vi "fromFiles.vi"(0 "MagAnalysis_Online in":refnum<class "MagAnalysis_Online.lvclass">, 1 "SubscriberCluster":T1, 2 "Clibration":T7, 5 "Images":T6, 7 "BGImages":T3, 9 "data":T5, 11 "error in (no error)":errorcluster, 12 "Numeric 3":i32) -> (3 "OK":bool[](array[boolean]), 4 "MagAnalysis_Online out":refnum<class "MagAnalysis_Online.lvclass">, 6 "ROI":T11, 8 "new ROI":bool, 10 "spec cluster":cluster{dbl[], dbl[]}, 13 "Numeric 2":u32, 14 "change from file":dbl, 15 "Numeric":dbl)   [LabVIEW 2011, in "MagAnalysis_Online.lvclass"]
uses:
  MagAnalysis_Online.lvclass
  SubVis/ROIStartfromCam_typdef.ctl
  SubVis/ScreenCam_TypDEf.ctl
  SubVis/ROIInfo_TypDef.ctl
  calib_Sub_Typdef.ctl
  Calib_Typdef.ctl
  <vilib>/vision/Image Controls.llb/IMAQ Image.ctl
  analysis_data_typdef.ctl
  SubVis/dataTypdef.ctl
  bgImages_tyudef.ctl
  Interface/GUI_Template/GUI_master/tcp new data cluster.ctl
  Interface/GUI_Template/GUI_master/tcp_new_data_event.ctl
  shared/SubscriberCluster_TypDEf.ctl
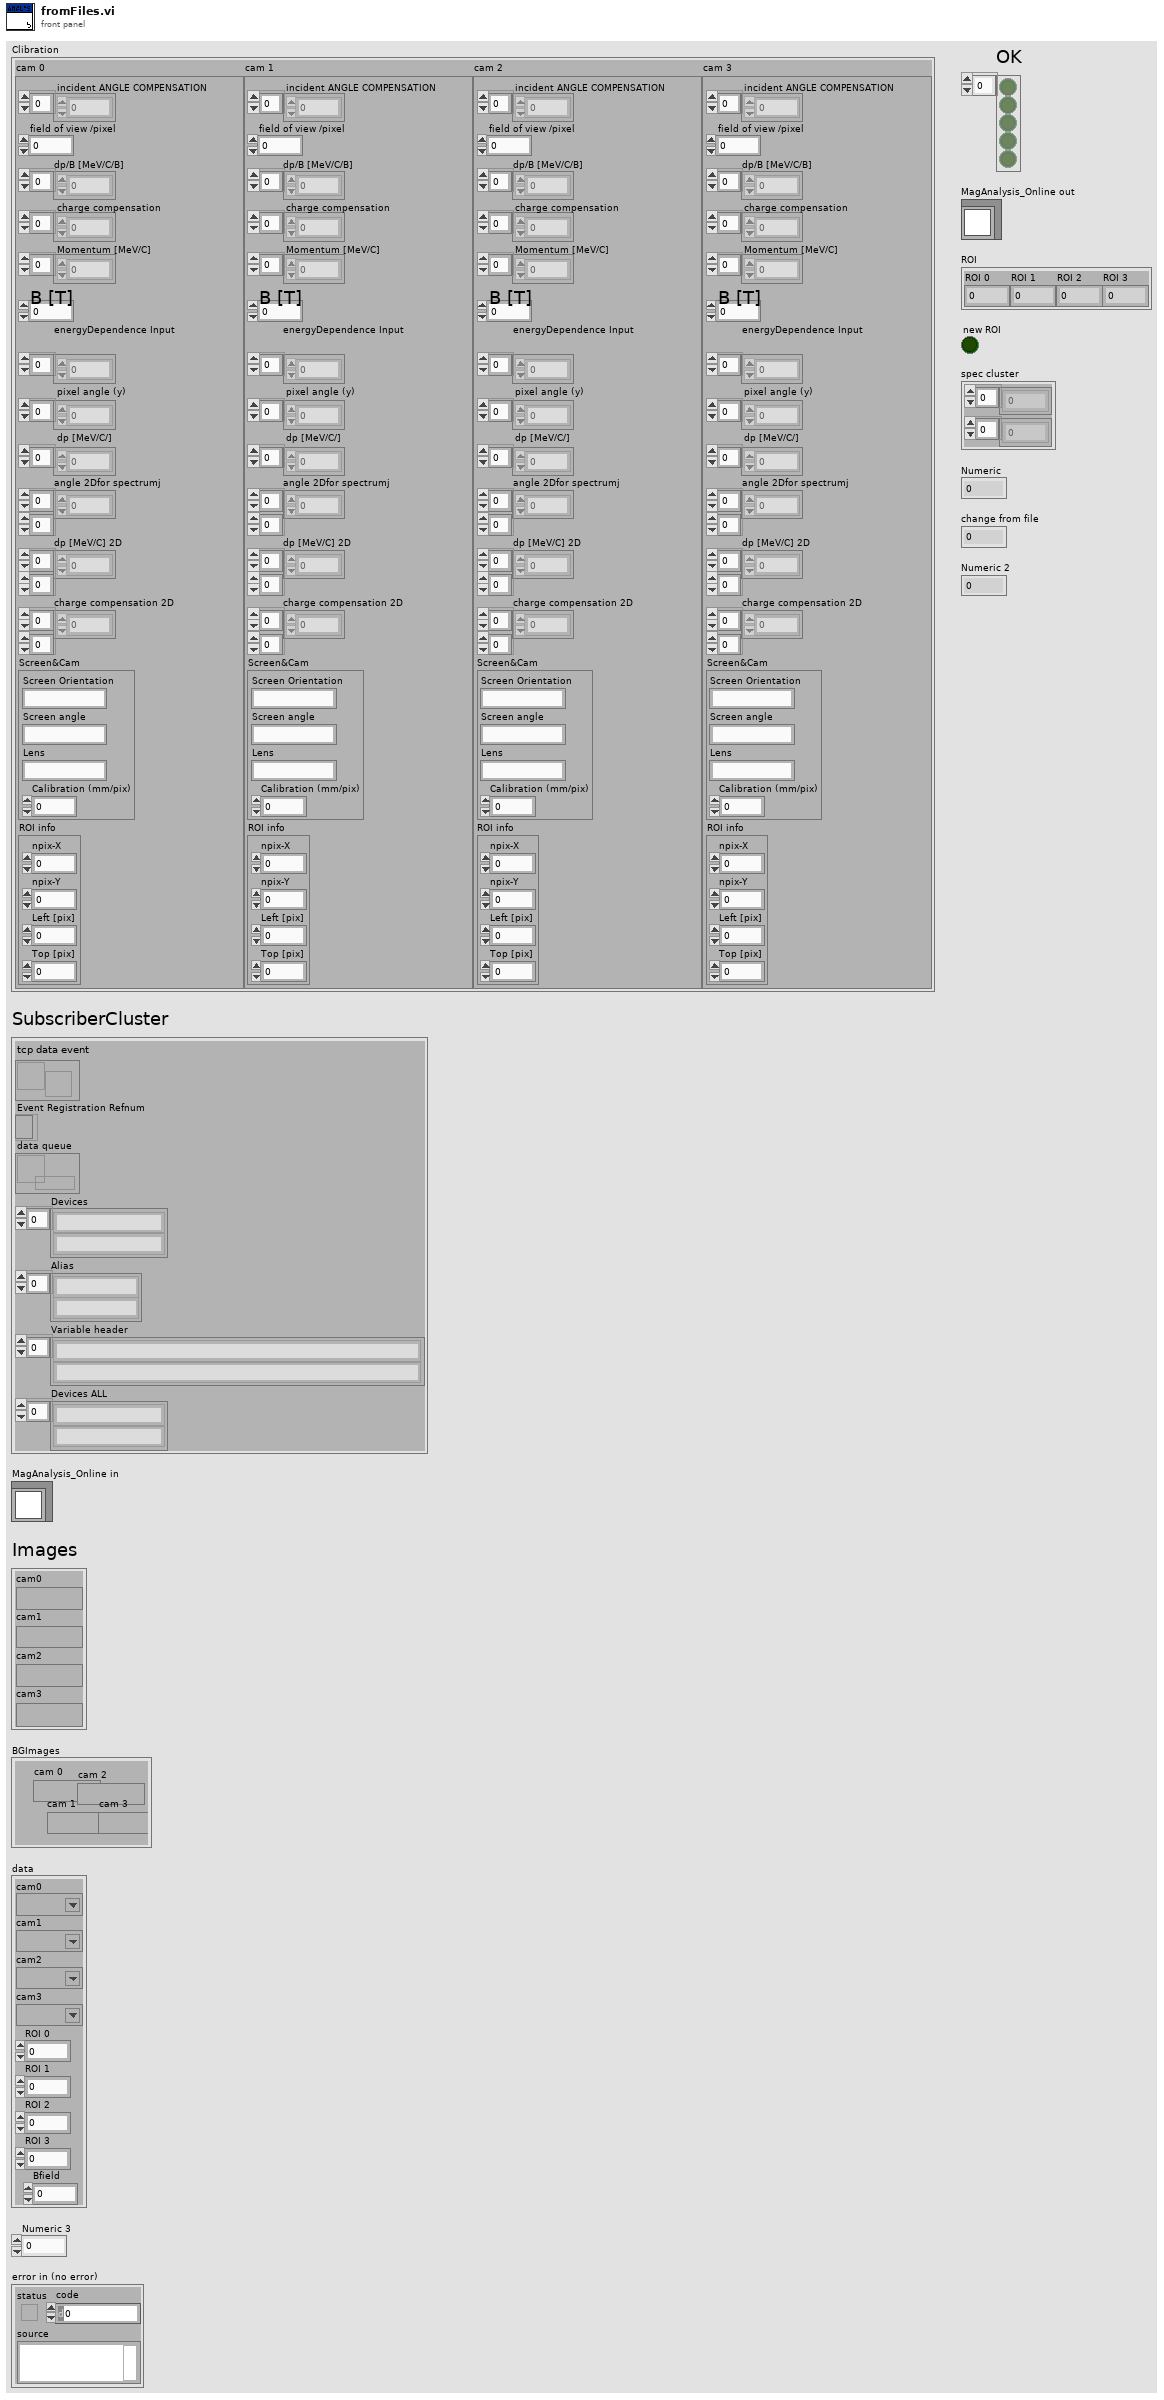
[diagram p1: front panel]
types:
  T1 = typedef "SubscriberCluster_TypDEf.ctl" = cluster{"tcp data event":T2, "Event Registration Refnum":refnum<event-registration>, "data queue":refnum<queue>, "Devices":string[], "Alias":string[], "Variable header":string[], "Devices ALL":string[]}
  T2 = typedef "tcp_new_data_event.ctl" = refnum<user-event>
  T3 = typedef "bgImages_tyudef.ctl" = cluster{"cam 0":T4, "cam 1":T4, "cam 2":T4, "cam 3":T4}
  T4 = typedef "IMAQ Image.ctl" = refnum<image>
  T5 = typedef "dataTypdef.ctl" = cluster{"cam0":T4, "cam1":T4, "cam2":T4, "cam3":T4, "ROI 0":dbl, "ROI 1":dbl, "ROI 2":dbl, "ROI 3":dbl, "Bfield":dbl}
  T6 = typedef "MagAnalysis_Online.lvclass/analysis_data_typdef.ctl" = cluster{"cam0":T4, "cam1":T4, "cam2":T4, "cam3":T4}
  T7 = typedef "Calib_Typdef.ctl" = cluster{"cam 0":T8, "cam 1":T8, "cam 2":T8, "cam 3":T8}
  T8 = typedef "calib_Sub_Typdef.ctl" = cluster{"incident ANGLE COMPENSATION":dbl[], "field of view /pixel":dbl, "dp/B [MeV/C/B]":dbl[], "charge compensation":dbl[], "Momentum [MeV/C]":dbl[], "B [T]":dbl, "energyDependence Input":dbl[], "pixel angle (y)":dbl[], "dp [MeV/C/] ":dbl[], "angle 2Dfor spectrumj":dbl[][], "dp [MeV/C] 2D":dbl[][], "charge compensation 2D":dbl[][], "Screen&Cam":T9, "ROI info":T10}
  T9 = typedef "ScreenCam_TypDEf.ctl" = cluster{"Screen Orientation":string, "Screen angle":string, "Lens":string, "Calibration (mm/pix)":dbl}
  T10 = typedef "ROIInfo_TypDef.ctl" = cluster{"npix-X":i32, "npix-Y":i32, "Left [pix]":dbl, "Top [pix]":dbl}
  T11 = typedef "ROIStartfromCam_typdef.ctl" = cluster{"ROI 0":dbl, "ROI 1":dbl, "ROI 2":dbl, "ROI 3":dbl}
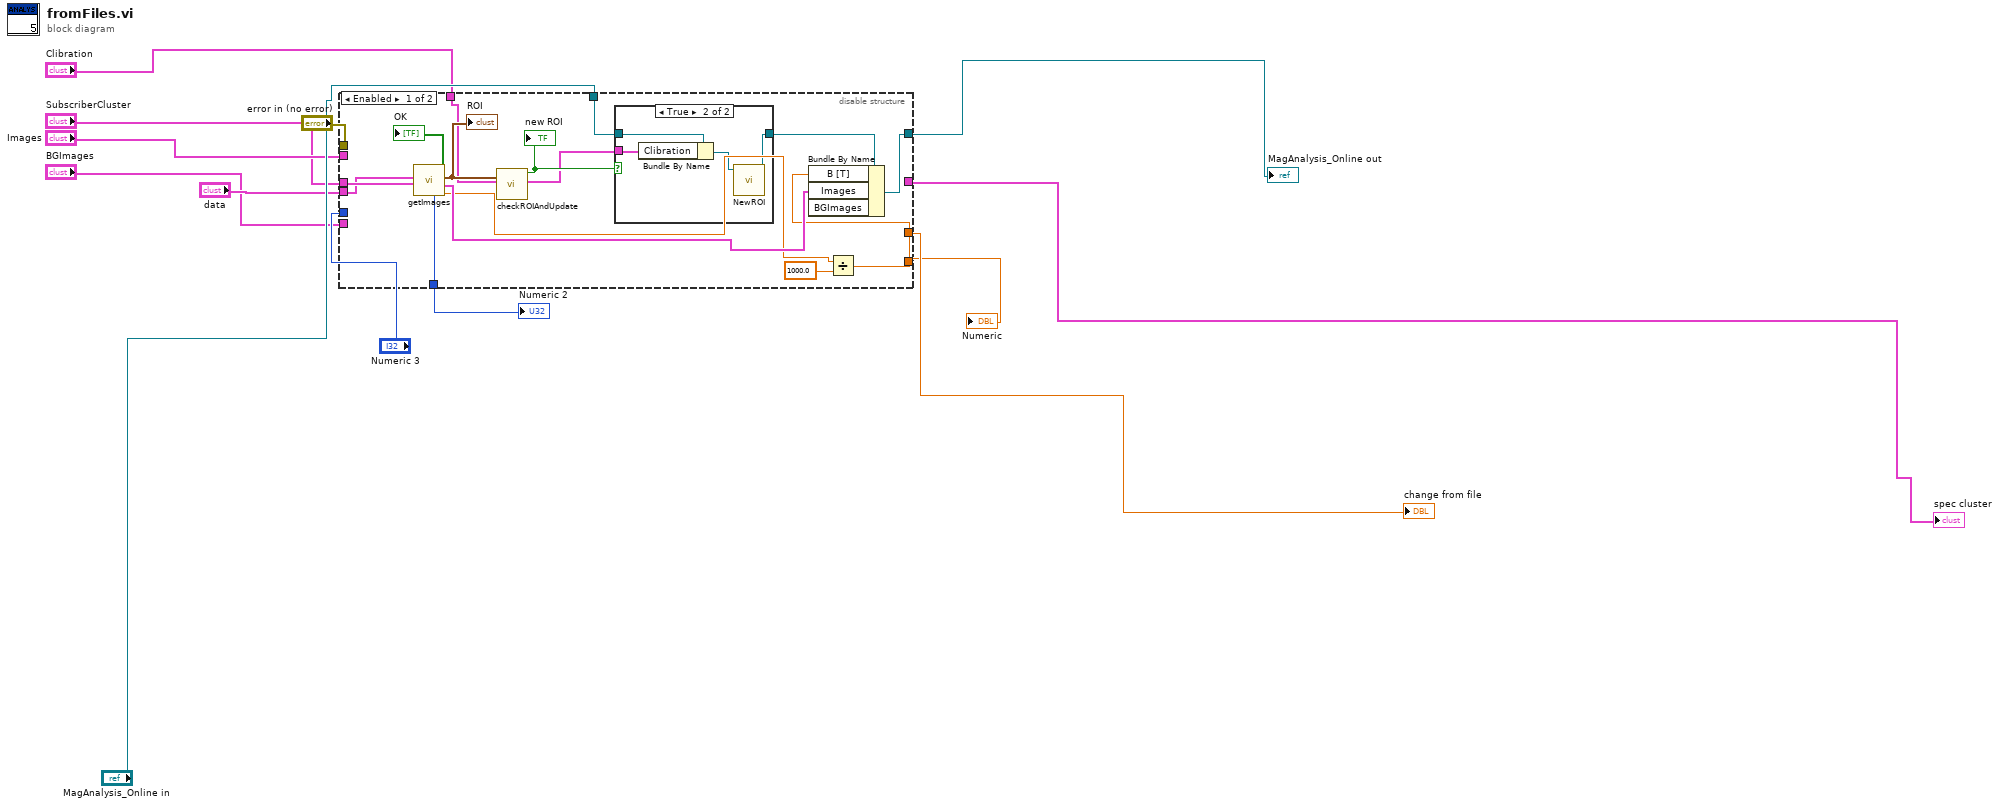
[diagram p0: block diagram]
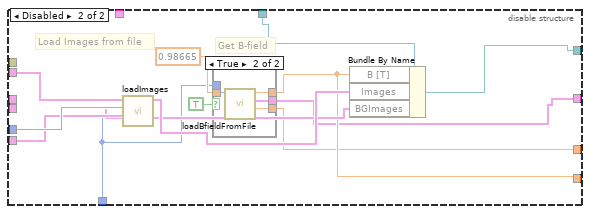
[diagram p3: hidden frame]
diagram:
  n1 = disable-structure shown="Enabled" {
    disable-tunnel: "SubscriberCluster" -> [w28 _]
    disable-tunnel: "data" -> [w27 _]
    disable-tunnel: "Numeric 3" -> [_ w46]
    disable-tunnel: "error in (no error)" -> [_ _]
    disable-tunnel: "BGImages" -> [_ w45]
    disable-tunnel: "Images" -> [_ w44]
    disable-tunnel: [w26 w38] -> w7
    disable-tunnel: "Clibration" -> [w23 _]
    disable-tunnel: "MagAnalysis_Online in" -> [w20 w43]
    disable-tunnel: [w15 w37] -> w10
    disable-tunnel: [w14 w36] -> w11
    disable-tunnel: [_ w35] -> w12
    disable-tunnel: [_ w34] -> w13
    frame Enabled {
      n2 = call "getImages.vi"("data"=w27, "SubscriberCluster"=w28) -> ("B[mT]"=w17:dbl, "Images"=w19:T6, "ROI"=w24:T11, "OK"=→"OK":bool[], "Numeric"=w26:u32)  [unwired: 5 in]
      "ROI" <- w24
      n3 = call "checkROIAndUpdate.vi"("Clibration"=w23, "ROI in"=w24) -> ("Clibration out"=w21:cluster{"[0]":T8, "[1]":T8, "[2]":T8, "[3]":T8}, "new ROI"=w22:bool)  [unwired: 8 in]
      "new ROI" <- w22
      n4 = case shown="True" w22 {
        tunnel: w21 -> [_ w33]
        tunnel: w20 -> [w29 w32]
        tunnel: [w29 w30] -> w16
        frame False {
        }
        frame True {
          n5 = Bundle By Name(cluster=w32, "Clibration"=w33) -> (w31:refnum<class "MagAnalysis_Online.lvclass">)
          n6 = call "NewROI.vi"("MagAnalysis_Online in"=w31) -> ("MagAnalysis_Online out"=w30:refnum<class "MagAnalysis_Online.lvclass">)  [unwired: 10 in]
        }
      }
      n7 = Divide(x=w17, y=1000.0) -> (x/y=w14:dbl)
      n8 = Bundle By Name(cluster=w16, "B [T]"=w14, "Images"=w19) -> (w15:refnum<class "MagAnalysis_Online.lvclass">)  [unwired: 1 in]
    }
    frame Disabled {
      # "Get B-field"
      # "Load Images from file"
      n9 = call "loadImages.vi"("BGImages"=w45, "Numeric"=w46, "data"=w44) -> ("time"=w38:u32, "BG Images out"=w41:T3, "dat6a out"=w42:T6)  [unwired: 6 in]
      n10 = case shown="True" TRUE {
        tunnel: [w47 w51] -> w36
        tunnel: 0.98665 ("B [T] 2") -> [w47 _]
        tunnel: [_ w50] -> w34
        tunnel: w38 -> [_ w49]
        tunnel: [_ w48] -> w35
        frame False {
        }
        frame True {
          n11 = call "loadBfieldFromFile.vi"("index"=w49) -> ("change from file"=w48:dbl, "spec cluster"=w50:cluster{dbl[], dbl[]}, "B [T]"=w51:dbl)  [unwired: 8 in]
        }
      }
      n12 = Bundle By Name(cluster=w43, "B [T]"=w36, "Images"=w42, "BGImages"=w41) -> (w37:refnum<class "MagAnalysis_Online.lvclass">)
    }
  }
  "spec cluster" <- w13
  "change from file" <- w12
  "Numeric" <- w11
  "MagAnalysis_Online out" <- w10
  "Numeric 2" <- w7
